vi "arange (SubVI).vi"(9 "# Steps":i32, 10 "stop":ext, 11 "start":ext) -> (3 "Array":ext[](array[numeric]))   [LabVIEW 2014]
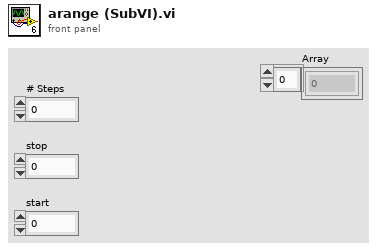
[diagram p1: front panel]
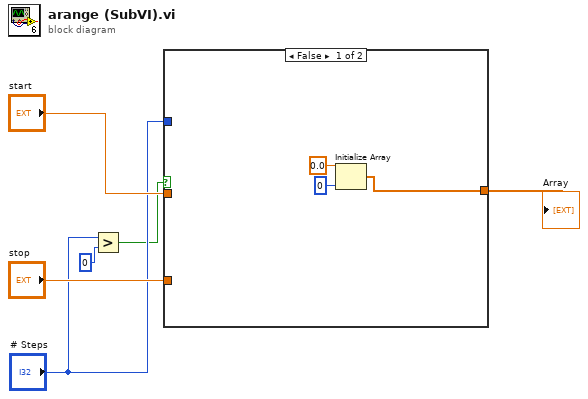
[diagram p0: block diagram]
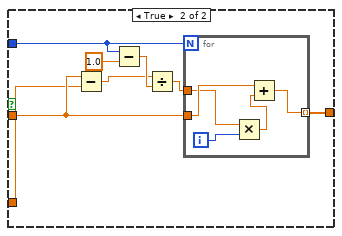
[diagram p2: hidden frame]
diagram:
  n1 = Greater?(x="# Steps", y=0) -> (0:w1:bool)
  n2 = case shown="False" w1 {
    tunnel: "# Steps" -> [_ w14]
    tunnel: "start" -> [_ w12]
    tunnel: "stop" -> [_ w11]
    tunnel: [w9 w10] -> w4
    frame False {
      n3 = Initialize Array(0.0 ("element"), 0 ("dimension size")) -> (w9:dbl[])
    }
    frame True {
      n4 = Subtract(x=w12, y=w11) -> (x-y=w13:ext)
      n5 = Subtract(x=w14, y=1.0) -> (x-y=w16:dbl)
      n6 = Divide(x=w13, y=w16) -> (x/y=w17:ext)
      n7 = for {
        N: w14 -> [_]
        tunnel: w12 -> [w22]
        tunnel: [w21] -> w10 mode=indexing
        tunnel: w17 -> [w18]
        i -> [w20]
        n8 = Multiply(x=w18, y=w20) -> (x*y=w19:ext)
        n9 = Add(x=w22, y=w19) -> (x+y=w21:ext)
      }
    }
  }
  "Array" <- w4
